vi "Ic_Complex_combination.vi"(10 "2D array in 2":u8[][](array[numeric]), 11 "2D array in":u8[][](array[numeric])) -> (3 "2D array out":u8[][](array[numeric]))   [LabVIEW 2014]
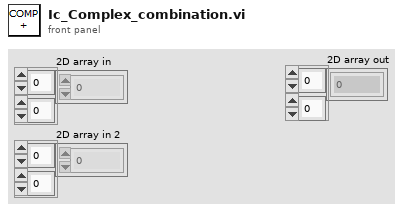
[diagram p1: front panel]
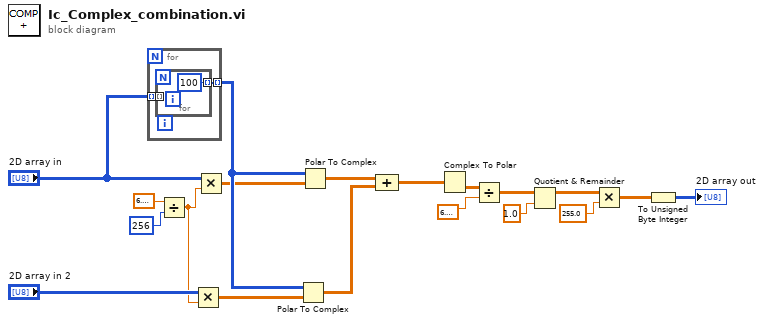
[diagram p0: block diagram]
diagram:
  n1 = for {
    tunnel: "2D array in" -> [w21] mode=indexing
    tunnel: [w20] -> w11 mode=indexing
    n2 = for {
      tunnel: w21 -> [_] mode=indexing
      tunnel: [100] -> w20 mode=indexing
    }
  }
  n3 = Divide(x=6.283185307179586, y=u16 256) -> (x/y=w10:dbl)
  n4 = Multiply(x="2D array in 2", y=w10) -> (x*y=w12:dbl[][])
  n5 = Multiply(x="2D array in", y=w10) -> (x*y=w2:dbl[][])
  n6 = Polar To Complex(1:w12, 2:w11) -> (0:w8:cdb[][])
  n7 = Polar To Complex(1:w2, 2:w11) -> (0:w9:cdb[][])
  n8 = Compound Arithmetic op=ADD(w9, w8) -> (w1:cdb[][])
  n9 = Complex To Polar(r * e^(i*theta)=w1) -> (theta=w14:dbl[][])  [unwired: 1 out]
  n10 = Divide(x=w14, y=6.283185307179586) -> (x/y=w4:dbl[][])
  n11 = Quotient & Remainder(x=w4, y=1.0) -> (x-y*floor(x/y)=w7:dbl[][])  [unwired: 1 out]
  n12 = Multiply(x=w7, y=255.0) -> (x*y=w3:dbl[][])
  n13 = To Unsigned Byte Integer(number=w3) -> (unsigned 8bit integer=→"2D array out":u8[][])
